vi "Version.vi"(8 "error in (no error)":errorcluster, 11 "S4GUI in":refnum<class "S4GUI.lvclass">) -> (0 "error out":errorcluster, 3 "S4GUI out":refnum<class "S4GUI.lvclass">)   [LabVIEW 2018, in "S4GUI.lvclass"]
uses:
  S4GUI.lvclass
  S4GUI.lvclass/S4GUI.ctl
  Log/Log.lvclass
  SyncBox/Sync Box.lvclass
  Acquisition/Acquisition.lvclass
  Instrument/Instrument.lvclass
  TCS/TCS.lvclass
  TelFocus/TelFocus.lvclass
  WeatherStation/WeatherStation.lvclass
  GSserver/GSserver.lvclass
  Publisher/Publisher.lvclass
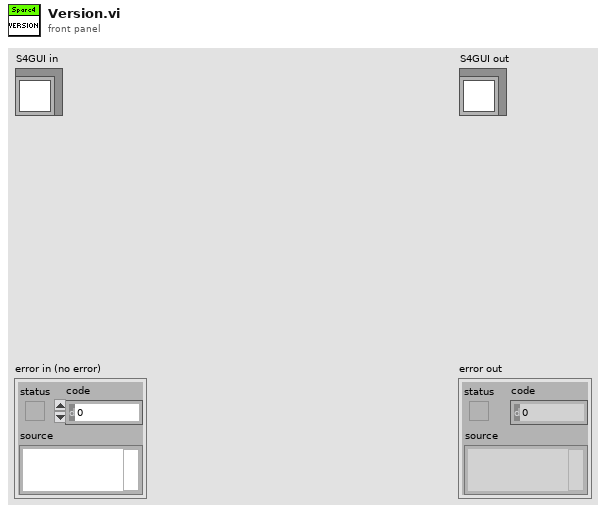
[diagram p1: front panel]
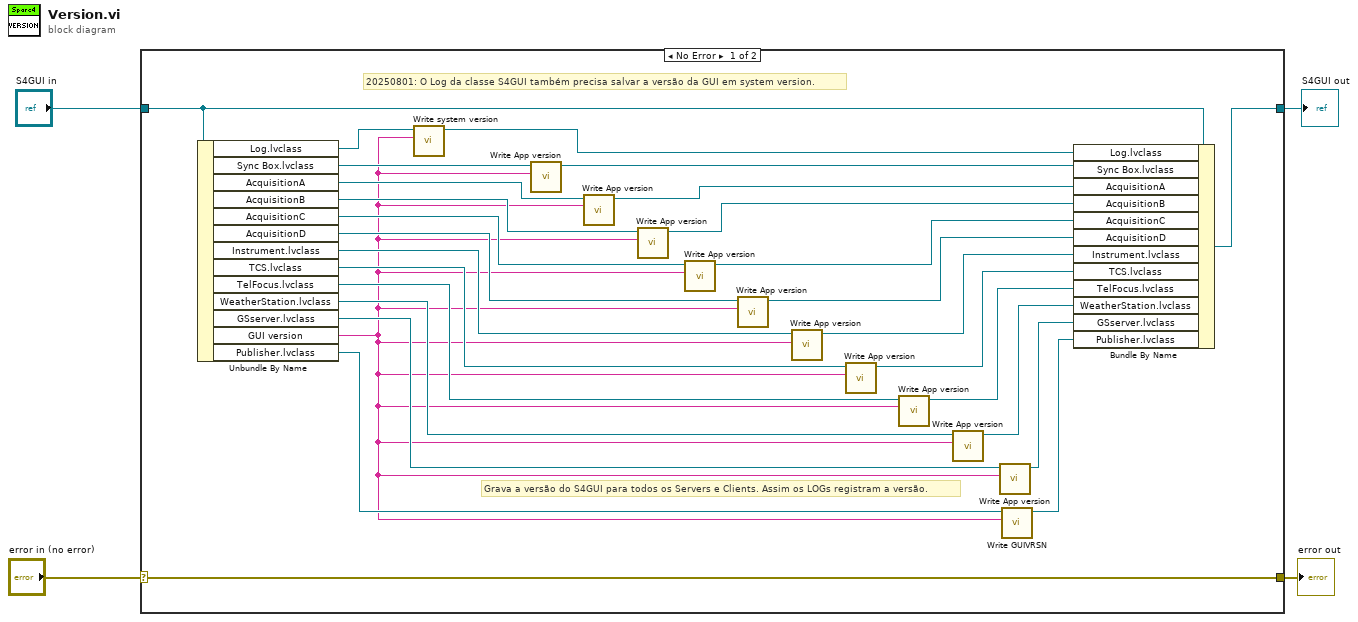
[diagram p0: block diagram]
diagram:
  n1 = case shown="No Error" "error in (no error)" {
    selector: "error in (no error)" -> [w32 w34]
    tunnel: [w32 w34] -> w3
    tunnel: [w20 w33] -> w1
    tunnel: "S4GUI in" -> [w21 w33]
    frame No Error {
      # "20250801: O Log da classe S4GUI também precisa salvar a versão da GUI em system version."
      # "Grava a versão do S4GUI para todos os Servers e Clients. Assim os LOGs registram a versão."
      n2 = Unbundle By Name(w21) -> ("Log.lvclass"=w9:refnum<class "Log.lvclass">, "Sync Box.lvclass"=w31:refnum<class "Sync Box.lvclass">, "AcquisitionA"=w30:refnum<class "Acquisition.lvclass">, "AcquisitionB"=w29:refnum<class "Acquisition.lvclass">, "AcquisitionC"=w28:refnum<class "Acquisition.lvclass">, "AcquisitionD"=w27:refnum<class "Acquisition.lvclass">, "Instrument.lvclass"=w26:refnum<class "Instrument.lvclass">, "TCS.lvclass"=w25:refnum<class "TCS.lvclass">, "TelFocus.lvclass"=w24:refnum<class "TelFocus.lvclass">, "WeatherStation.lvclass"=w23:refnum<class "WeatherStation.lvclass">, "GSserver.lvclass"=w22:refnum<class "GSserver.lvclass">, "GUI version"=w5:string, "Publisher.lvclass"=w6:refnum<class "Publisher.lvclass">)
      n3 = call-dynamic "Write system version.vi"("system version"=w5, "Log in"=w9) -> ("Log out"=w8:refnum<class "Log.lvclass">)  [unwired: 8 in, 1 out]
      n4 = call-dynamic "Write App version.vi"("App version"=w5, "Server in"=w31) -> ("Server out"=w14:refnum<class "Sync Box.lvclass">)  [unwired: 8 in, 1 out]
      n5 = call-dynamic "Write App version.vi"("App version"=w5, "Server in"=w30) -> ("Server out"=w13:refnum<class "Acquisition.lvclass">)  [unwired: 8 in, 1 out]
      n6 = call-dynamic "Write App version.vi"("App version"=w5, "Server in"=w29) -> ("Server out"=w12:refnum<class "Acquisition.lvclass">)  [unwired: 8 in, 1 out]
      n7 = call-dynamic "Write App version.vi"("App version"=w5, "Server in"=w28) -> ("Server out"=w11:refnum<class "Acquisition.lvclass">)  [unwired: 8 in, 1 out]
      n8 = call-dynamic "Write App version.vi"("App version"=w5, "Server in"=w27) -> ("Server out"=w10:refnum<class "Acquisition.lvclass">)  [unwired: 8 in, 1 out]
      n9 = call-dynamic "Write App version.vi"("App version"=w5, "Server in"=w26) -> ("Server out"=w15:refnum<class "Instrument.lvclass">)  [unwired: 8 in, 1 out]
      n10 = call-dynamic "Write App version.vi"("App version"=w5, "Server in"=w25) -> ("Server out"=w16:refnum<class "TCS.lvclass">)  [unwired: 8 in, 1 out]
      n11 = call-dynamic "Write App version.vi"("App version"=w5, "Server in"=w24) -> ("Server out"=w17:refnum<class "TelFocus.lvclass">)  [unwired: 8 in, 1 out]
      n12 = call-dynamic "Write App version.vi"("App version"=w5, "Server in"=w23) -> ("Server out"=w18:refnum<class "WeatherStation.lvclass">)  [unwired: 8 in, 1 out]
      n13 = call-dynamic "Write App version.vi"("App version"=w5, "Server in"=w22) -> ("Server out"=w19:refnum<class "GSserver.lvclass">)  [unwired: 8 in, 1 out]
      n14 = call-dynamic "Write GUIVRSN.vi"("GUIVRSN"=w5, "Publisher in"=w6) -> ("Publisher out"=w7:refnum<class "Publisher.lvclass">)  [unwired: 8 in, 1 out]
      n15 = Bundle By Name(cluster=w21, "Log.lvclass"=w8, "Sync Box.lvclass"=w14, "AcquisitionA"=w13, "AcquisitionB"=w12, "AcquisitionC"=w11, "AcquisitionD"=w10, "Instrument.lvclass"=w15, "TCS.lvclass"=w16, "TelFocus.lvclass"=w17, "WeatherStation.lvclass"=w18, "GSserver.lvclass"=w19, "Publisher.lvclass"=w7) -> (w20:refnum<class "S4GUI.lvclass">)
    }
    frame Error {
    }
  }
  "error out" <- w3
  "S4GUI out" <- w1
